vi "Encode -decode One Time Pad.vi"(5 "Pad":string="\u000f0\u0004YXXXXgGFw6%!@@YsstttgF677HHEII4s&CtYP\u0007\u0007ivhXv))HHes44CVUhXyw\u0007XHIYVYIIiXC8IYYVXHHiDTTTC444CA\u0004Y\u0000\u0000\u0003C3\u0004", 6 "error in (no error)":errorcluster, 9 "Text in":string="abcdefghijklmnopqrstuvwxyz") -> (0 "error out":errorcluster, 3 "Text out":string)   [LabVIEW 2012]
doc: "This vi will convert encrypted text to un-encrypted and vice versa using the one time pad method. If the \"pad' text string is not wired the default front panel value is used. Note- this vi automatatically encodes or decodes text (actions are symetric).\n\nNote - if the text in is longer than the pad the pad is extended (by a custom algoirthm) until it is long enough to encode or decode the text.\n\nIf error in = T text out = text in."
panel:
  # "hex display"
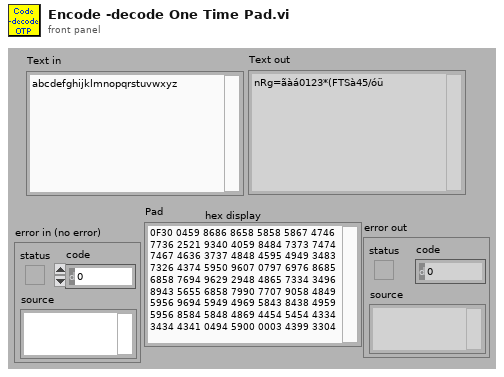
[diagram p1: front panel]
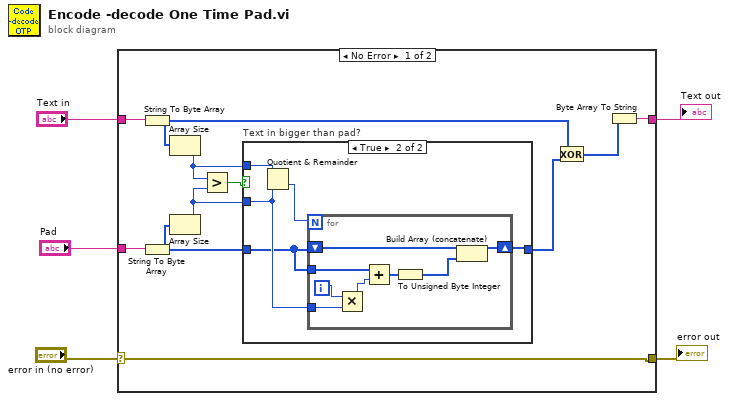
[diagram p0: block diagram]
diagram:
  n1 = case shown="No Error" "error in (no error)" {
    selector: "error in (no error)" -> [w16 w32]
    tunnel: [w16 w32] -> w4
    tunnel: [w9 w31] -> w2
    tunnel: "Text in" -> [w15 w31]
    tunnel: "Pad" -> [w14 _]
    frame No Error {
      n2 = String To Byte Array(string=w15) -> (unsigned byte array=w13:u8[])
      n3 = String To Byte Array(string=w14) -> (unsigned byte array=w12:u8[])
      n4 = Array Size(array=w13) -> (size(s)=w7:i32)
      n5 = Array Size(array=w12) -> (size(s)=w6:i32)
      n6 = Greater?(x=w7, y=w6) -> (0:w11:bool)
      n7 = case "Text in bigger than pad?" shown="True" w11 {
        tunnel: [w17 w18] -> w8
        tunnel: w12 -> [w17 w19]
        tunnel: w7 -> [_ w22]
        tunnel: w6 -> [_ w20]
        frame False {
        }
        frame True {
          n8 = Quotient & Remainder(x=w22, y=w20) -> (floor(x/y)=w21:i32)  [unwired: 1 out]
          n9 = for {
            N: w21 -> [_]
            shift-right: [w25] -> w18
            shift-left: w19 -> [w27]
            tunnel: w20 -> [w30]
            tunnel: w19 -> [w24]
            i -> [w29]
            n10 = Multiply(x=w29, y=w30) -> (x*y=w28:i32)
            n11 = Add(x=w24, y=w28) -> (x+y=w26:i32[])
            n12 = To Unsigned Byte Integer(number=w26) -> (unsigned 8bit integer=w23:u8[])
            n13 = Build Array (concatenate)(w27, w23) -> (w25:u8[])
          }
        }
      }
      n14 = Exclusive Or(1:w8, 2:w13) -> (0:w10:u8[])
      n15 = Byte Array To String(unsigned byte array=w10) -> (string=w9:string)
    }
    frame Error {
    }
  }
  "Text out" <- w2
  "error out" <- w4
